vi "GlobalFileFind.vi"(9 "GlobalVariableArray 2":cluster{"name":string, "va;":dbl}[](array[cluster])=[{"name"="Val1", "va;"=1.0}, {"name"="Val2", "va;"=2.0}, {"name"="Val3", "va;"=3.0}, {"name"="Val4", "va;"=4.0}], 10 "VariableNameLookup":string) -> (2 "VariableValueOut":dbl)   [LabVIEW 2011]
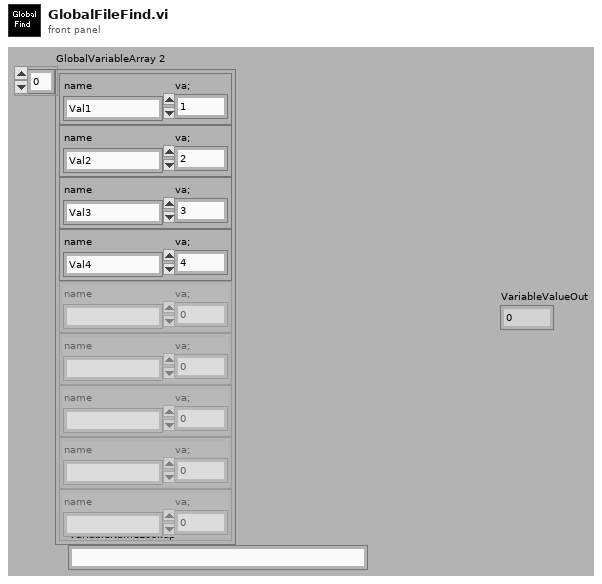
[diagram p1: front panel]
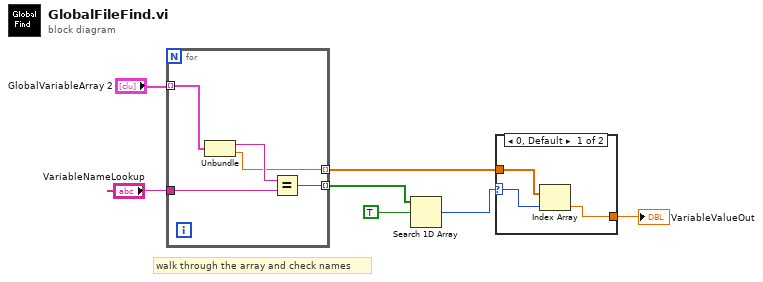
[diagram p0: block diagram]
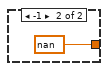
[diagram p2: hidden frame]
diagram:
  # "walk through the array and check names"
  n1 = for {
    tunnel: "GlobalVariableArray 2" -> [w12] mode=indexing
    tunnel: "VariableNameLookup" -> [w10]
    tunnel: [w9] -> w7 mode=indexing
    tunnel: [w8] -> w4 mode=indexing
    n2 = Unbundle(w12) -> ("name"=w11:string, "va;"=w8:dbl)
    n3 = Equal?(x=w11, y=w10) -> (x = y?=w9:bool)
  }
  n4 = Search 1D Array(1D array=w7, element=TRUE) -> (index of element=w5:i32)  [unwired: 1 out]
  n5 = case shown="0, Default" w5 {
    selector: w5 -> [w14 _]
    tunnel: [w13 nan ("Value")] -> w2
    tunnel: w4 -> [w15 _]
    frame 0, Default {
      n6 = Index Array(array=w15, index=w14) -> (element=w13:dbl)
    }
    frame -1 {
    }
  }
  "VariableValueOut" <- w2
